vi "无效产品.vi"   [LabVIEW 2017]
panel:
  # "当前选择的产品型号有误\n请检查产品型号是否符合规范"
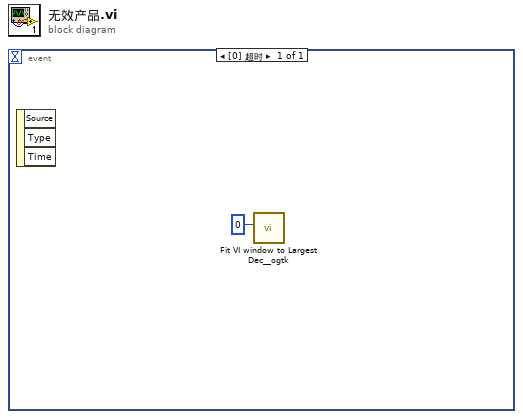
[diagram p0: block diagram]
diagram:
  n1 = event shown="[0] 超时" {
    selector: _ -> [_]
    dyn-events: _ -> [_]
    timeout: _ -> [_]
    event Timeout {
      n2 = event-data() -> ()  [unwired: 1 in, 3 out]
      n3 = call <userlib>:"Fit VI window to Largest Dec__ogtk.vi"("border spacing (2 px)"=0) -> ()  [unwired: 5 in, 2 out]
    }
  }
